vi "LoadDateProfileWrapper.vi"(8 "error in (no error)":errorcluster, 11 "PatientDatePath":path) -> (0 "error out":errorcluster, 3 "profile":T1)   [LabVIEW 2013, in "main.lvlib"]
uses:
  main.lvlib
  <userlib>/_OpenG.lib/file/file.llb/File Exists - Scalar__ogtk.vi
  <vilib>/Utility/file.llb/Read From Spreadsheet File (string).vi
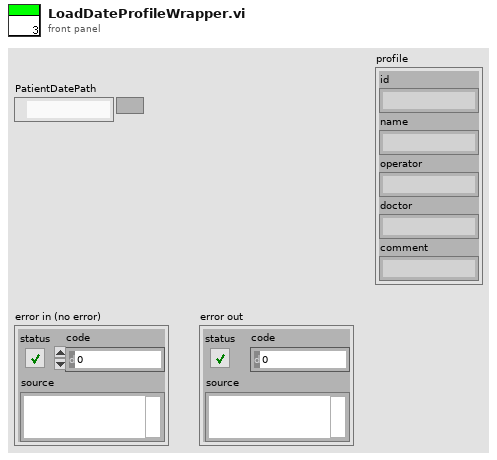
[diagram p1: front panel]
types:
  T1 = cluster{"id":string, "name":string, "operator":string, "doctor":string, "comment":string}
  T2 = cluster{"String":string, "String":string, "String":string, "String":string, "String":string}
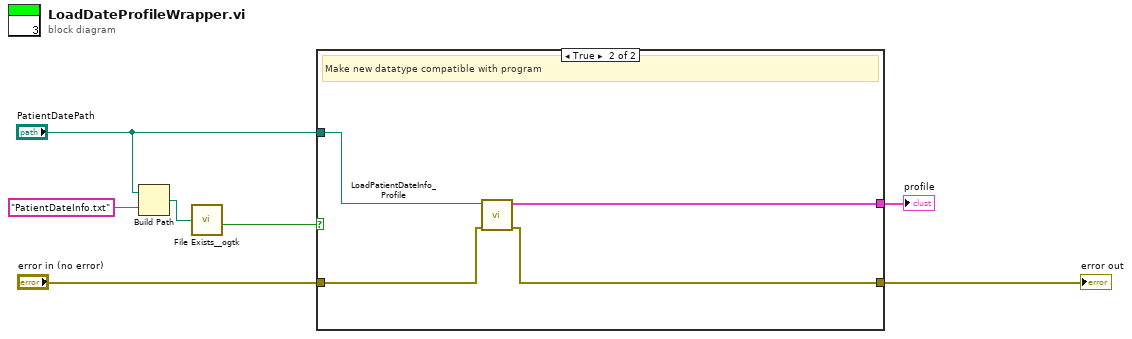
[diagram p0: block diagram]
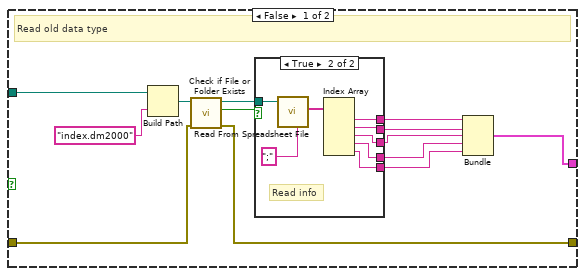
[diagram p2: hidden frame]
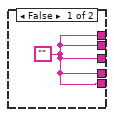
[diagram p3: hidden frame]
diagram:
  n1 = Build Path(base path="PatientDatePath", name or relative path="PatientDateInfo.txt") -> (appended path=w3:path)
  n2 = call-poly <userlib>:"File Exists__ogtk.vi"("file path"=w3) -> ("exists"=w2:bool)  [unwired: 6 in, 1 out]
  n3 = case shown="True" w2 {
    tunnel: [w20 w32] -> w7
    tunnel: "error in (no error)" -> [w19 w33]
    tunnel: "PatientDatePath" -> [w14 w30]
    tunnel: [w8 w31] -> w1
    frame False {
      # "Read old data type"
      n4 = Build Path(base path=w14, name or relative path="index.dm2000") -> (appended path=w16:path)
      n5 = call <vilib>:"Check if File or Folder Exists.vi"("error in (no error)"=w19, "path"=w16) -> ("error out"=w20:errorcluster, "file or folder exists?"=w18:bool, "dup path"=w17:path)  [unwired: 7 in]
      n6 = case shown="True" w18 {
        tunnel: w17 -> [_ w29]
        tunnel: [w21 w26] -> w12
        tunnel: [w21 w25] -> w11
        tunnel: [w21 w24] -> w10
        tunnel: [w21 w23] -> w9
        tunnel: [w21 w22] -> w13
        frame False {
          w21 = ""
        }
        frame True {
          # "Read info"
          n7 = call-poly <vilib>:"Read From Spreadsheet File.vi"("delimiter (\\t)"=";" ("delimiter (\\t)"), "file path (dialog if empty)"=w29) -> ("first row"=w28:string[])  [unwired: 5 in, 4 out]
          n8 = Index Array(array=w28) -> (element #1=w22:string, element #2=w26:string, element #3=w25:string, element #4=w24:string, element #5=w23:string)  [unwired: 5 in]
        }
      }
      n9 = Bundle("String"=w13, "String"=w12, "String"=w11, "String"=w10, "String"=w9) -> (w8:T2)  [unwired: 1 in]
    }
    frame True {
      # "Make new datatype compatible with program"
      n10 = call "LoadPatientDateInfo_Profile.vi"("error in"=w33, "DataPatientDatePath"=w30) -> ("error out"=w32:errorcluster, "profile"=w31:T1)  [unwired: 8 in]
    }
  }
  "error out" <- w7
  "profile" <- w1
